vi "Intan_SDcardConfig.vi"(0 "VISA resource name":refnum<visa-resource-name>="COM1", 1 "SdFilename":string, 2 "error in":errorcluster, 3 "FileSize(MB)":i16) -> (4 "error out":errorcluster, 5 "Return File Name":string, 6 "VISA resource name out":refnum<visa-resource-name>, 7 "Sd init string":string, 8 "SDCardResultStr":string, 9 "ErrorOpeningSDfile":bool)   [LabVIEW 2017]
panel:
  out "CreateContigFileResult":string
  out "ReqFileSzString":string
  out "Request Filename":string
  in  "Teensy event char":string="d"
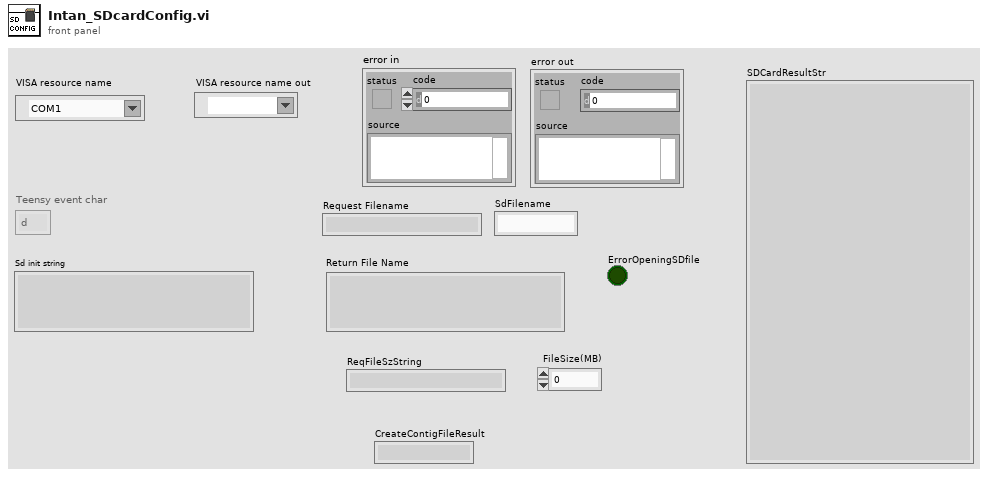
[diagram p1: front panel]
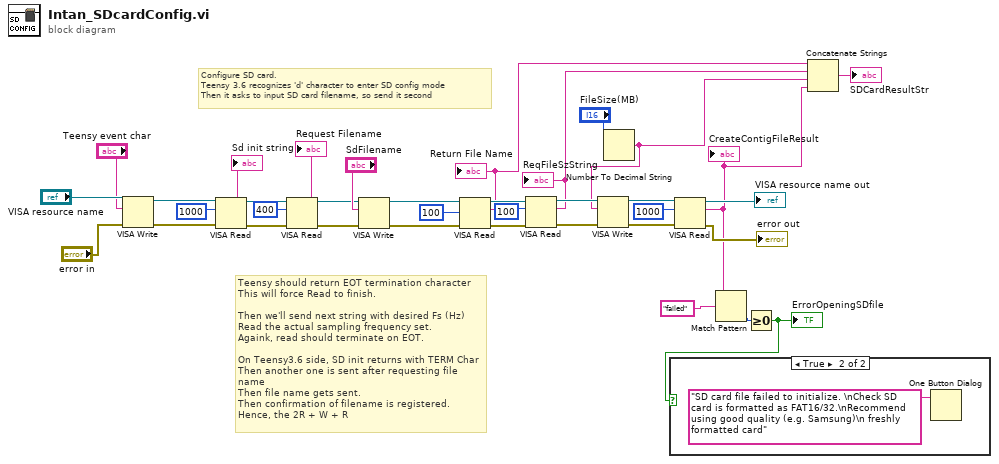
[diagram p0: block diagram]
diagram:
  # "Configure SD card. \nTeensy 3.6 recognizes 'd' character to enter SD config mode\nThen it asks to input SD card filename, so send it second"
  # "Teensy should return EOT termination character \nThis will force Read to finish.\n\nThen we'll send next string with desired Fs (Hz)\nRead the actual sampling frequency set.\nAgaink, read should terminate on EOT.\n\nOn Teensy3.6 side, SD init returns with TERM Char\nThen another one is sent after requesting file name\nThen file name gets sent.\nThen confirmation of filename is registered.\nHence, the 2R + W + R"
  n1 = VISA Write(VISA resource name="VISA resource name", write buffer="Teensy event char", error in (no error)="error in") -> (VISA resource name out=w31:refnum<visa-resource-name>, error out=w30:errorcluster)  [unwired: 1 out]
  n2 = VISA Read(VISA resource name=w31, byte count=u32 1000, error in (no error)=w30) -> (VISA resource name out=w25:refnum<visa-resource-name>, read buffer=→"Sd init string":string, error out=w23:errorcluster)  [unwired: 1 out]
  n3 = VISA Read(VISA resource name=w25, byte count=u32 400, error in (no error)=w23) -> (VISA resource name out=w24:refnum<visa-resource-name>, read buffer=→"Request Filename":string, error out=w22:errorcluster)  [unwired: 1 out]
  n4 = VISA Write(VISA resource name=w24, write buffer="SdFilename", error in (no error)=w22) -> (VISA resource name out=w28:refnum<visa-resource-name>, error out=w27:errorcluster)  [unwired: 1 out]
  n5 = VISA Read(VISA resource name=w28, byte count=u32 100, error in (no error)=w27) -> (VISA resource name out=w14:refnum<visa-resource-name>, read buffer=w5:string, error out=w13:errorcluster)  [unwired: 1 out]
  "Return File Name" <- w5
  n6 = VISA Read(VISA resource name=w14, byte count=u32 100, error in (no error)=w13) -> (VISA resource name out=w16:refnum<visa-resource-name>, read buffer=w4:string, error out=w15:errorcluster)  [unwired: 1 out]
  "ReqFileSzString" <- w4
  n7 = Number To Decimal String(number="FileSize(MB)") -> (decimal integer string=w3:string)  [unwired: 1 in]
  n8 = VISA Write(VISA resource name=w16, write buffer=w3, error in (no error)=w15) -> (VISA resource name out=w10:refnum<visa-resource-name>, error out=w9:errorcluster)  [unwired: 1 out]
  n9 = VISA Read(VISA resource name=w10, byte count=u32 1000, error in (no error)=w9) -> (VISA resource name out=→"VISA resource name out":refnum<visa-resource-name>, read buffer=w2:string, error out=→"error out":errorcluster)  [unwired: 1 out]
  "CreateContigFileResult" <- w2
  n10 = Match Pattern(string=w2, regular expression="failed") -> (offset past match=w18:i32)  [unwired: 1 in, 3 out]
  n11 = Greater Or Equal To 0?(x=w18) -> (x >= 0?=w17:bool)
  "ErrorOpeningSDfile" <- w17
  n12 = case shown="True" w17 {
    frame False {
    }
    frame True {
      n13 = One Button Dialog(message="SD card file failed to initialize. \nCheck SD card is formatted as FAT16/32.\nRecommend using good quality (e.g. Samsung)\n freshly formatted card") -> ()  [unwired: 1 in, 1 out]
    }
  }
  n14 = Concatenate Strings(w5, w4, w3, w2) -> (→"SDCardResultStr":string)
